vi "StopMods.vi"(8 "ErrorArray":errorcluster[](array[cluster]), 11 "TestBase in":refnum<class "TestBase.lvclass">) -> (0 "ErrorArray":errorcluster[](array[cluster]), 3 "TestBase out":refnum<class "TestBase.lvclass">)   [LabVIEW 2014, in "TestBase.lvclass"]
uses:
  TestBase.lvclass
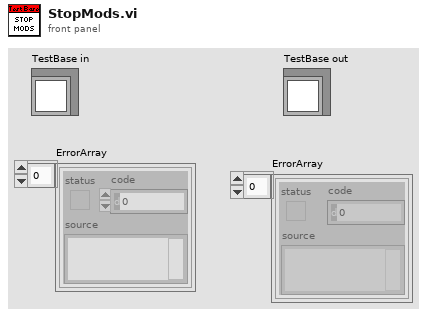
[diagram p1: front panel]
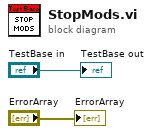
[diagram p0: block diagram]
diagram:
  "TestBase out" <- "TestBase in"
  "ErrorArray" <- "ErrorArray"
